vi "Create_Path.vi"(8 "error in":errorcluster, 10 "Extension":string=".xlsx", 11 "Saving parameters":T1={"Path on the output file"=path "D:/Programmation/Labview_ILM_LIDT/DATA", "Filename without extension"="Measurement_1"}) -> (0 "error out":errorcluster, 3 "File path":path=path "D:/Programmation/Labview_ILM_LIDT/DATA/Measurement_1.xlsx")   [LabVIEW 2023]
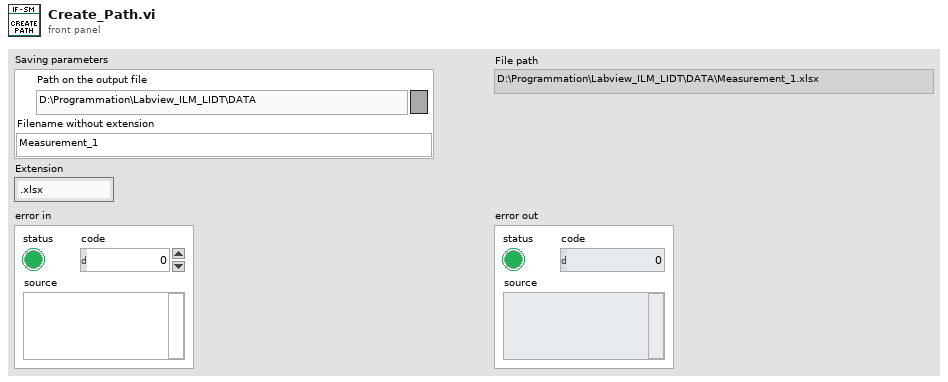
[diagram p1: front panel]
types:
  T1 = cluster{"Path on the output file":path, "Filename without extension":string}
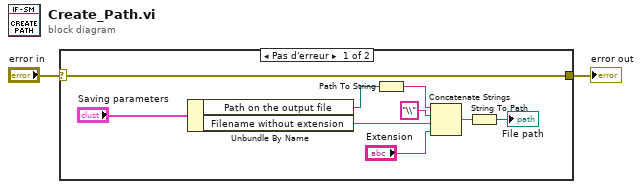
[diagram p0: block diagram]
diagram:
  n1 = case shown="Pas d'erreur" "error in" {
    selector: "error in" -> [w11 w12]
    tunnel: [w11 w12] -> w1
    frame No Error {
      n2 = Unbundle By Name("Saving parameters") -> ("Path on the output file"=w9:path, "Filename without extension"=w6:string)
      n3 = Path To String(path=w9) -> (string=w8:string)
      n4 = Concatenate Strings(w8, "\\", w6, "Extension") -> (w5:string)
      n5 = String To Path(string=w5) -> (path=→"File path":path)
    }
    frame Error {
    }
  }
  "error out" <- w1
